vi "Data Logger Main.vi"(0 "WebDAV Push":bool, 1 "In Spec":bool[](array[boolean])=[FALSE, FALSE, FALSE, FALSE, FALSE, FALSE], 2 "Current Step":i32=2, 3 "Step Time Left":dbl=0.21101045608520508, 4 "Pump Data":T2={"Voltages"=[0.015201568603515625, 0.00335693359375, 0.003021240234375, 0.12260055541992188, 0.06085968017578125, 0.052234649658203125], "PumpCurrent"=[0.015201568603515625, 0.00335693359375, 0.003021240234375, 0.12260055541992188, 0.06085968017578125, 0.052234649658203125], "Speed"=[0.0, 0.0, 0.0, 0.0, 0.0, 0.0], "ControllerCurrent"=[0.015201568603515625, 0.00335693359375, 0.003021240234375, 0.12260055541992188, 0.06085968017578125, 0.052234649658203125], "Pressure"=[0.015201568603515625, 0.00335693359375, 0.003021240234375, 0.12260055541992188, 0.06085968017578125, 0.052234649658203125], "Flow"=[0.0, 0.0, 0.0, 0.125, 0.0625, 0.0625], "Elapsed Time (Display)"=[7.1, 7.1, 7.1, 458133.45, 458138.85000000003, 458126.75], "Avg Pressure"=0.0, "Avg Speed"=0.0, "Elapsed Time"=[4074.9003000000002, 4074.9003000000002, 4074.9003000000002, 4074.9003000000002, 4074.9003000000002, 4074.9003000000002]} {"Elapsed Time" format="%<%H:%M:%S>t"; "Elapsed Time (Display)" format="%<%H:%M:%S>t"; "Speed" format="%#_4f"; "ControllerCurrent" format="%#.1g"; "Pressure" format="%#.0f"; "Flow" format="%#.0f"; "PumpCurrent" format="%#.1g"; "Voltages" format="%#.0f"}, 5 "Tank Data":T1 {"PS Actual (V):" format="%.2f"; "Temp1" format="%#_2g"; "Temp2" format="%#_2g"}, 6 "Concat Data":bool, 7 "Record Time (sec)":dbl, 8 "Data Logger Mode":T8=enum."Main", 9 "Data Log Start":T3={"App Config"={"Location"="", "Profiles Path"=path "", "Current Profile"="", "CA Number"="", "Cycles Completed"=0, "Controller Type:"=enum."Kuhnke", "Stagger Time (ms)"=0, "Tank 1 Fuel"="", "Tank 2 Fuel"="", "Serial Numbers"={"Position 1 SN"="", "Position 2 SN"="", "Poaition 3 SN"="", "Position 4 SN"="", "Position 5 SN"="", "Position 6 SN"=""}, "Pumps Present"={"Pump 1"=FALSE, "Pump 2"=FALSE, "Pump 3"=FALSE, "Pump 4"=FALSE, "Pump 5"=FALSE, "Pump 6"=FALSE}, "VoltCtrlRef"="", "VoltageSelect"=FALSE, "Watlow Present"=FALSE, "Temp 1"=0.0, "Temp 2"=0.0, "V_Run PI?"=FALSE, "Voltage Limits"={"V_Step"=1e-05, "V_CmdMax"=0.0, "V_CmdMin"=0.0}, "Voltage Far PI"={"V_FarSlew"=10.0, "V_FarKp"=0.0, "V_FarKi"=0.0}, "Voltage Mid PI"={"V_MidSlew"=10.0, "V_MidKp"=0.0, "V_MidKi"=0.0}, "Voltage Close PI"={"V_CloseSlew"=10.0, "V_CloseKp"=0.0, "V_CloseKi"=0.0}, "Voltage Scale"={"V_FFm"=0.0, "V_FFb"=0.0}, "Voltage Cutoffs"={"V_MidCutoff"=0.0, "V_CloseCutoff"=0.0}, "Pressure Scale"={"Pres_FFm"=1e-05, "Pres_FFb"=0.0}, "Temp Format"=0, "Temp Tolerance"=0.0, "Target Voltage"=0.0, "Target Pressure"=0.0, "Data Log Init"={"Data Path"=path "", "Data Log Rate (S/s)"=0, "AKLH Rate (Hours/S)"=0.0, "Sync Time Offset (min)"=0, "IP Last 3"=0, "WebDAV IP"=""}, "Email Handler IP"="", "ADC Check"=FALSE, "3 Pump Tank"=FALSE, "Cycle Threshold:"=3.0, "Cycle Pts to Avg:"=3, "Anomaly Threshold:"=3.0, "Normal Steps:"=3, "Step Threshold:"=3.0, "Network Drive IP"="", "Network Drive Password"="", "Bank 1 Offset"=0.0, "Bank 2 Offset"=0.0}, "Profile"=[], "Controller Type"="", "Tank CMDs"={"PS CMD"=0.0, "Press CMD"=0.0, "Temp 1 CMD"=0.0, "Temp 2 CMD"=0.0}} {"App Config"."Bank 2 Offset" min=0.0 max=999999.0 step=1.0; "App Config"."Bank 1 Offset" min=0.0 max=999999.0 step=1.0; "App Config"."Step Threshold:" min=0.0 max=999999.0 step=1.0; "App Config"."Normal Steps:" max=999999 step=1; "App Config"."Anomaly Threshold:" min=0.0 max=999999.0 step=1.0; "App Config"."Cycle Pts to Avg:" max=999999 step=1; "App Config"."Cycle Threshold:" min=0.0 max=999999.0 step=1.0}, 11 "Data Log Init":T6) -> ()   [LabVIEW 2013]
uses:
  Data Logger Mode.ctl
  Data Log Init.ctl
  Data Log Start.ctl
  Type Defs/App Config.ctl
  Type Defs/Controller Names.ctl
  Controls/Tank CMDs.ctl
  Controls/Pump Data.ctl
  Controls/Tank Data.ctl
  <userlib>/_OpenG.lib/array/array.llb/Remove Duplicates from 1D Array (String)__ogtk.vi
  <userlib>/_OpenG.lib/array/array.llb/Filter 1D Array (String)__ogtk.vi
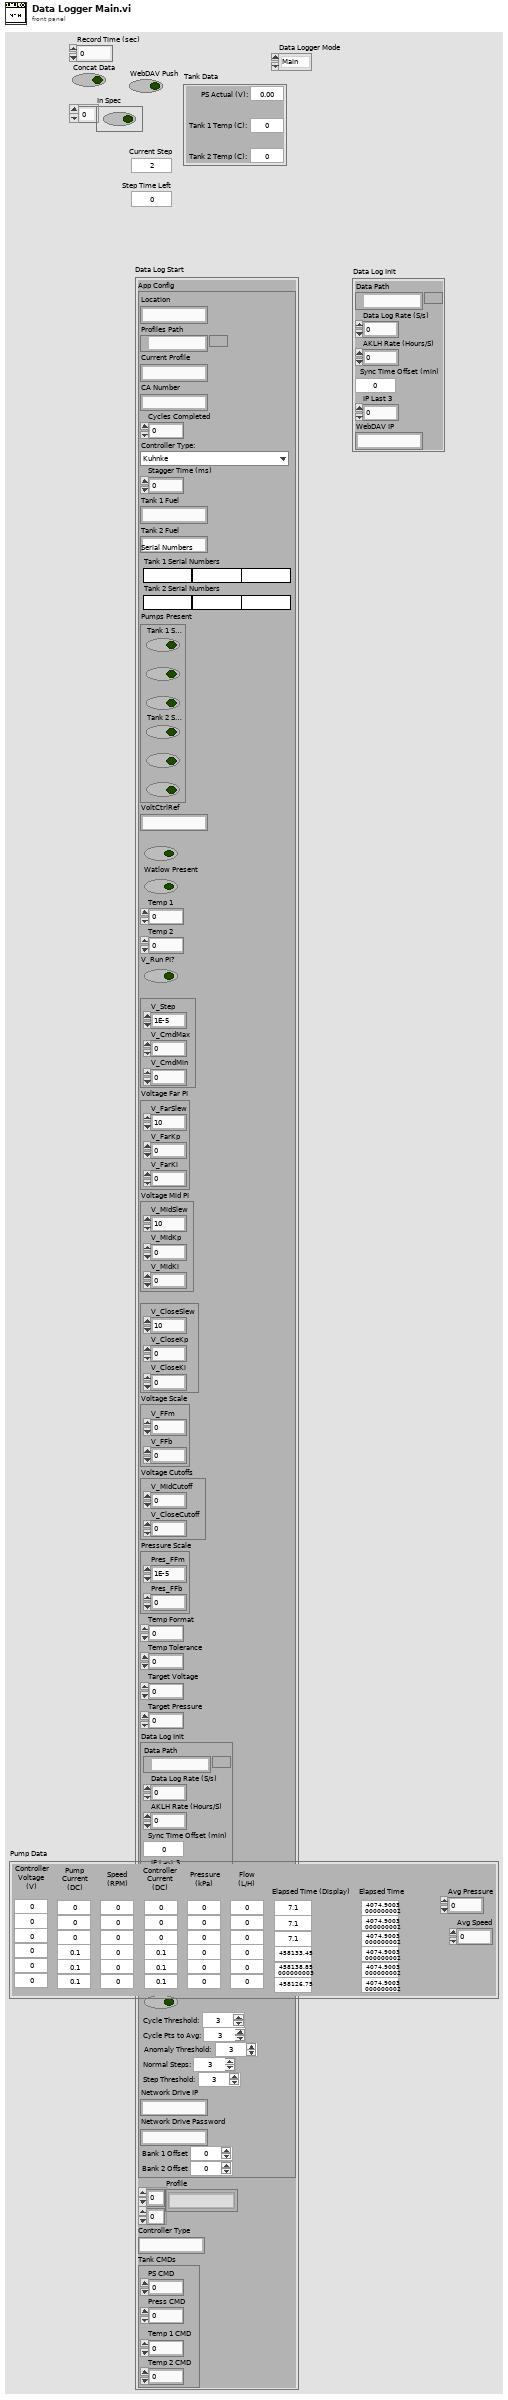
[diagram p1: front panel]
types:
  T1 = typedef "Tank Data.ctl" = cluster{"PS Actual (V):":dbl, "Temp1":dbl, "Temp2":dbl}
  T2 = typedef "Pump Data.ctl" = cluster{"Voltages":dbl[], "PumpCurrent":dbl[], "Speed":dbl[], "ControllerCurrent":dbl[], "Pressure":dbl[], "Flow":dbl[], "Elapsed Time (Display)":dbl[], "Avg Pressure":dbl, "Avg Speed":dbl, "Elapsed Time":dbl[]}
  T3 = typedef "Data Log Start.ctl" = cluster{"App Config":T4, "Profile":string[][], "Controller Type":string, "Tank CMDs":T7}
  T4 = typedef "App Config.ctl" = cluster{"Location":string, "Profiles Path":path, "Current Profile":string, "CA Number":string, "Cycles Completed":u32, "Controller Type:":T5, "Stagger Time (ms)":i32, "Tank 1 Fuel":string, "Tank 2 Fuel":string, "Serial Numbers":cluster{"Position 1 SN":string, "Position 2 SN":string, "Poaition 3 SN":string, "Position 4 SN":string, "Position 5 SN":string, "Position 6 SN":string}, "Pumps Present":cluster{"Pump 1":bool, "Pump 2":bool, "Pump 3":bool, "Pump 4":bool, "Pump 5":bool, "Pump 6":bool}, "VoltCtrlRef":string, "VoltageSelect":bool, "Watlow Present":bool, "Temp 1":dbl, "Temp 2":dbl, "V_Run PI?":bool, "Voltage Limits":cluster{"V_Step":dbl, "V_CmdMax":dbl, "V_CmdMin":dbl}, "Voltage Far PI":cluster{"V_FarSlew":dbl, "V_FarKp":dbl, "V_FarKi":dbl}, "Voltage Mid PI":cluster{"V_MidSlew":dbl, "V_MidKp":dbl, "V_MidKi":dbl}, "Voltage Close PI":cluster{"V_CloseSlew":dbl, "V_CloseKp":dbl, "V_CloseKi":dbl}, "Voltage Scale":cluster{"V_FFm":dbl, "V_FFb":dbl}, "Voltage Cutoffs":cluster{"V_MidCutoff":dbl, "V_CloseCutoff":dbl}, "Pressure Scale":cluster{"Pres_FFm":dbl, "Pres_FFb":dbl}, "Temp Format":i32, "Temp Tolerance":dbl, "Target Voltage":dbl, "Target Pressure":dbl, "Data Log Init":T6, "Email Handler IP":string, "ADC Check":bool, "3 Pump Tank":bool, "Cycle Threshold:":dbl, "Cycle Pts to Avg:":i32, "Anomaly Threshold:":dbl, "Normal Steps:":u32, "Step Threshold:":dbl, "Network Drive IP":string, "Network Drive Password":string, "Bank 1 Offset":dbl, "Bank 2 Offset":dbl}
  T5 = typedef "Controller Names.ctl" = enum16{"Kuhnke", "Helbako BLDC", "Conti", "Hella BLDC OL PWM", "Hella BLDC Turbine OL PWM", "Hella BLDC Pressure", "Helbako (old)", "TI PWM", "PSA", "Hella Gas", "Hella Diesel", "8 Comm", "10 Comm", "8 Comm Hella", "10 Comm Hella", "8 Comm Omron", "10 Comm Omron", "8 Comm Nissan", "10 Comm Nissan"}
  T6 = typedef "Data Log Init.ctl" = cluster{"Data Path":path, "Data Log Rate (S/s)":u32, "AKLH Rate (Hours/S)":dbl, "Sync Time Offset (min)":i32, "IP Last 3":i32, "WebDAV IP":string}
  T7 = typedef "Tank CMDs.ctl" = cluster{"PS CMD":dbl, "Press CMD":dbl, "Temp 1 CMD":dbl, "Temp 2 CMD":dbl}
  T8 = typedef "Data Logger Mode.ctl" = enum16{"Init", "Main", "Start", "Stop"}
  T9 = cluster{"Pump 1":bool, "Pump 2":bool, "Pump 3":bool, "Pump 4":bool, "Pump 5":bool, "Pump 6":bool}
  T10 = cluster{"Data Log Base":path, "AKLH Base":path, "AKLH Today Base":path, "AKLH Sync Base":path, "Data Log Rate (ms)":u32, "AKLH Rate (ms)":u32, "Sync Time (min)":i32, "Profile":string[][], "Target Speeds":string[], "App Config":T4, "AKLH Filenames":string[], "Data Log Dirs":path[], "AKLH Dirs":path[], "AKLH Today Dirs":path[], "AKLH Sync Dirs":path[], "Data Log Hdr Paths":path[], "AKLH Today Hdr Paths":path[], "Log Data":bool, "Data Log Times":u32[], "AKLH Log Times":u32[][], "WebDAV IP":string, "Tank CMDs":T7}
  T11 = cluster{"Position 1 SN":string, "Position 2 SN":string, "Poaition 3 SN":string, "Position 4 SN":string, "Position 5 SN":string, "Position 6 SN":string}
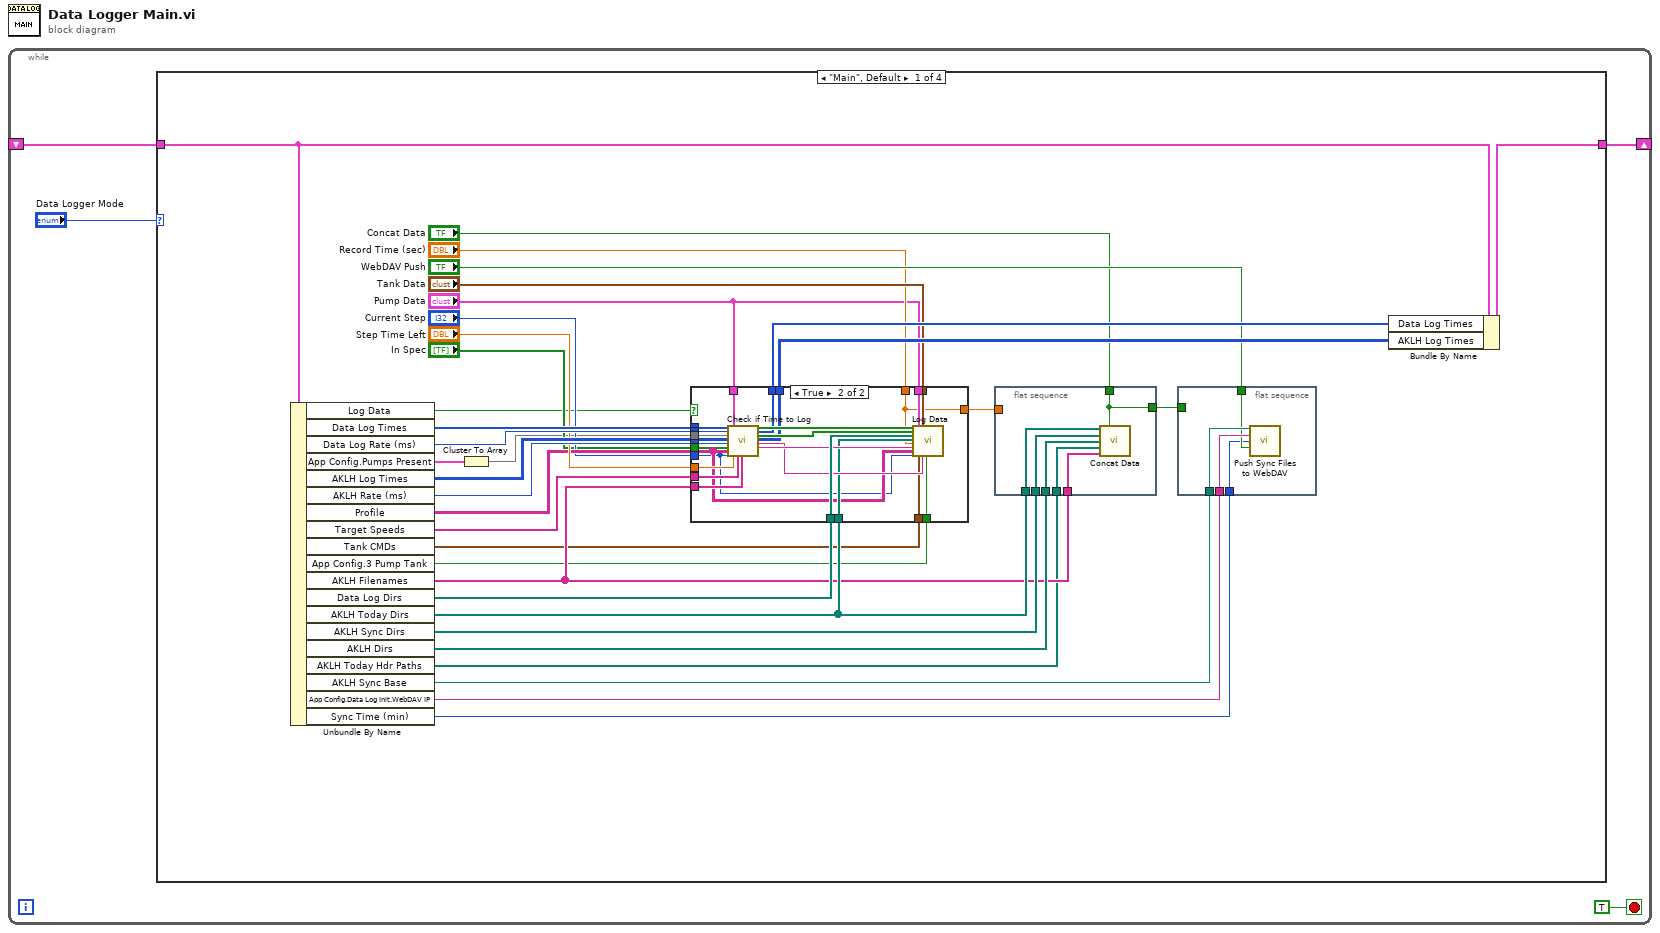
[diagram p0: block diagram]
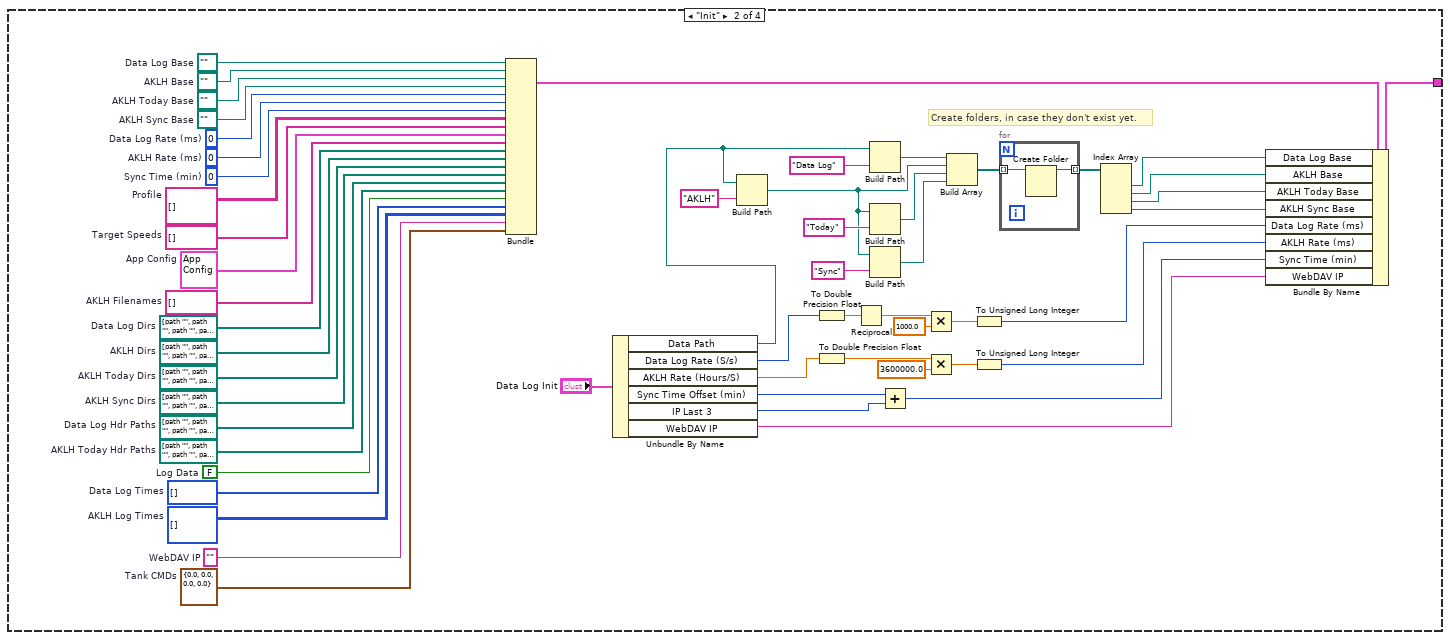
[diagram p3: hidden frame]
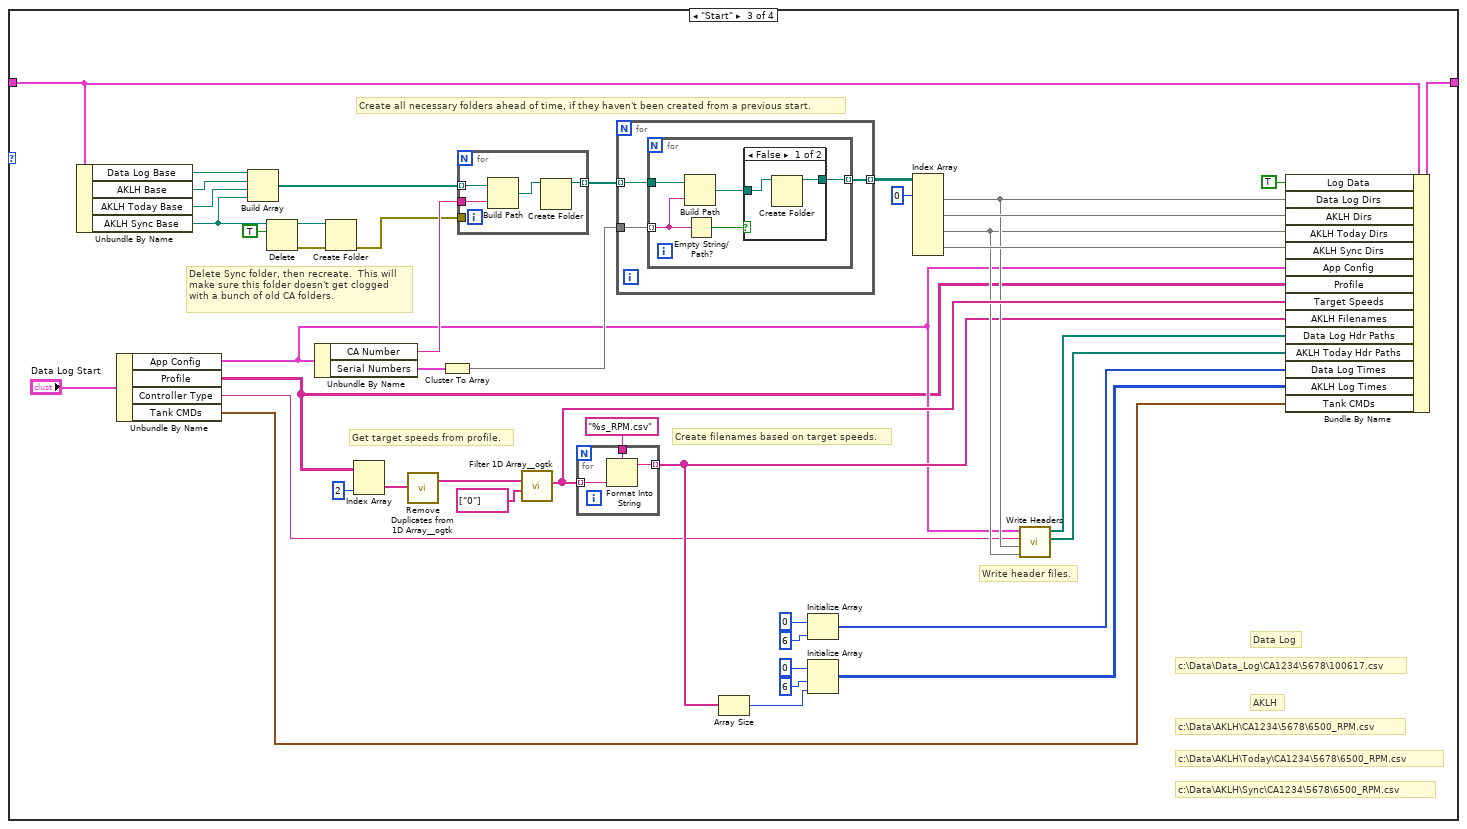
[diagram p4: hidden frame]
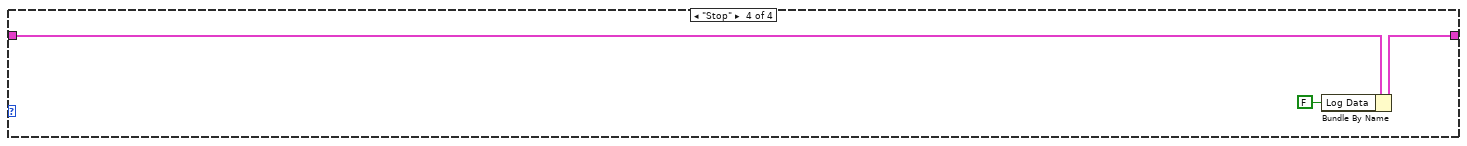
[diagram p6: hidden frame]
diagram:
  n1 = while {
    shift-right: [w2] -> _
    shift-left: _ -> [w1]
    stop <- TRUE stop-if-true
    n2 = case shown="\"Main\", Default" "Data Logger Mode" {
      tunnel: [w37 w124 w161 w196] -> w2
      tunnel: w1 -> [w38 _ w162 w197]
      frame "Main", Default {
        n3 = Unbundle By Name(w38) -> ("Log Data"=w9:bool, "Data Log Times"=w36:u32[], "Data Log Rate (ms)"=w35:u32, "App Config.Pumps Present"=w13:T9, "AKLH Log Times"=w34:u32[][], "AKLH Rate (ms)"=w33:u32, "Profile"=w18:string[][], "Target Speeds"=w31:string[], "Tank CMDs"=w16:T7, "App Config.3 Pump Tank"=w6:bool, "AKLH Filenames"=w24:string[], "Data Log Dirs"=w30:path[], "AKLH Today Dirs"=w27:path[], "AKLH Sync Dirs"=w26:path[], "AKLH Dirs"=w25:path[], "AKLH Today Hdr Paths"=w23:path[], "AKLH Sync Base"=w22:path, "App Config.Data Log Init.WebDAV IP"=w21:string, "Sync Time (min)"=w20:i32)
        n4 = Cluster To Array(cluster=w13) -> (array=w12:bool[])
        n5 = case shown="True" w9 {
          tunnel: w36 -> [w51 w76]
          tunnel: w35 -> [_ w75]
          tunnel: w34 -> [w50 w74]
          tunnel: w33 -> [_ w73]
          tunnel: "Step Time Left" -> [_ w72]
          tunnel: w31 -> [_ w71]
          tunnel: w30 -> [_ w68]
          tunnel: [w51 w65] -> w29
          tunnel: [w50 w64] -> w28
          tunnel: w27 -> [_ w63]
          tunnel: w24 -> [_ w62]
          tunnel: w18 -> [_ w56]
          tunnel: "Current Step" -> [_ w55]
          tunnel: w16 -> [_ w61]
          tunnel: "Tank Data" -> [_ w60]
          tunnel: "Pump Data" -> [_ w59]
          tunnel: "In Spec" -> [_ w58]
          tunnel: w12 -> [_ w57]
          tunnel: "Record Time (sec)" -> [w49 w54]
          tunnel: [w49 w54] -> w7
          tunnel: w6 -> [_ w53]
          tunnel: "Pump Data" -> [_ w52]
          frame False {
          }
          frame True {
            n6 = call "Check if Time to Log.vi"("Data Log Times IN"=w76, "Data Log Rate (ms)"=w75, "Pumps Present"=w57, "AKLH Log Times IN"=w74, "AKLH Rate (ms)"=w73, "In Spec"=w58, "Profile"=w56, "Current Step"=w55, "Pump Data"=w52, "Step Time Left"=w72, "Target Speeds"=w71, "AKLH Filenames"=w62) -> ("Log Data"=w70:bool[], "Data Log Times OUT"=w65:u32[], "Log AKLH"=w69:bool[], "AKLH Log Times OUT"=w64:u32[][], "AKLH Filename"=w66:string, "Target Speed"=w67:string)  [unwired: 10 in]
            n7 = call "Log Data.vi"("Log Data"=w70, "Log AKLH"=w69, "Data Log Dirs"=w68, "AKLH Today Dirs"=w63, "Record Time (sec)"=w54, "Target Speed"=w67, "Profile"=w56, "Current Step"=w55, "Pump Data"=w59, "Tank CMDs"=w61, "Tank Data"=w60, "AKLH Filename"=w66, "3 Pump Tank"=w53) -> ()  [unwired: 15 in]
          }
        }
        n8 = flat-sequence {
          tunnel: w27 -> [w48]
          tunnel: w26 -> [w47]
          tunnel: w25 -> [w46]
          tunnel: w24 -> [w45]
          tunnel: w23 -> [w44]
          tunnel: "Concat Data" -> [w43]
          tunnel: [w43] -> w8
          tunnel: w7 -> [_]
          frame #0 {
            n9 = call "Concat Data.vi"("AKLH Today Dirs"=w48, "Concat Data"=w43, "AKLH Sync Dirs"=w47, "AKLH Dirs"=w46, "AKLH Today Hdr Paths"=w44, "AKLH Filenames"=w45) -> ()  [unwired: 10 in]
          }
        }
        n10 = flat-sequence {
          tunnel: w22 -> [w42]
          tunnel: w21 -> [w41]
          tunnel: w20 -> [w39]
          tunnel: "WebDAV Push" -> [w40]
          tunnel: w8 -> [_]
          frame #0 {
            n11 = call "Push Sync Files to WebDAV.vi"("AKLH Sync Base"=w42, "WebDAV IP"=w41, "Sync Time (min)"=w39, "WebDAV Push"=w40) -> ()  [unwired: 12 in]
          }
        }
        n12 = Bundle By Name(cluster=w38, "Data Log Times"=w29, "AKLH Log Times"=w28) -> (w37:T10)
      }
      frame "Init" {
        w88 = T7 {"PS CMD"=0.0, "Press CMD"=0.0, "Temp 1 CMD"=0.0, "Temp 2 CMD"=0.0}  # Tank CMDs
        w94 = ""  # WebDAV IP
        w95 = u32[][] []  # AKLH Log Times
        w96 = u32[] []  # Data Log Times
        w97 = FALSE  # Log Data
        w98 = path[] [path "", path "", path "", path "", path "", path ""]  # AKLH Today Hdr Paths
        w99 = path[] [path "", path "", path "", path "", path "", path ""]  # Data Log Hdr Paths
        w100 = path[] [path "", path "", path "", path "", path "", path ""]  # AKLH Sync Dirs
        w101 = path[] [path "", path "", path "", path "", path "", path ""]  # AKLH Today Dirs
        w102 = path[] [path "", path "", path "", path "", path "", path ""]  # AKLH Dirs
        w103 = path[] [path "", path "", path "", path "", path "", path ""]  # Data Log Dirs
        w104 = string[] []  # AKLH Filenames
        w105 = T4 {"Location"="", "Profiles Path"=path "", "Current Profile"="", "CA Number"="", "Cycles Completed"=0, "Controller Type:"=enum."Kuhnke", "Stagger Time (ms)"=0, "Tank 1 Fuel"="", "Tank 2 Fuel"="", "Serial Numbers"={"Position 1 SN"="", "Position 2 SN"="", "Poaition 3 SN"="", "Position 4 SN"="", "Position 5 SN"="", "Position 6 SN"=""}, "Pumps Present"={"Pump 1"=FALSE, "Pump 2"=FALSE, "Pump 3"=FALSE, "Pump 4"=FALSE, "Pump 5"=FALSE, "Pump 6"=FALSE}, "VoltCtrlRef"="", "VoltageSelect"=FALSE, "Watlow Present"=FALSE, "Temp 1"=0.0, "Temp 2"=0.0, "V_Run PI?"=FALSE, "Voltage Limits"={"V_Step"=0.0, "V_CmdMax"=0.0, "V_CmdMin"=0.0}, "Voltage Far PI"={"V_FarSlew"=0.0, "V_FarKp"=0.0, "V_FarKi"=0.0}, "Voltage Mid PI"={"V_MidSlew"=0.0, "V_MidKp"=0.0, "V_MidKi"=0.0}, "Voltage Close PI"={"V_CloseSlew"=0.0, "V_CloseKp"=0.0, "V_CloseKi"=0.0}, "Voltage Scale"={"V_FFm"=0.0, "V_FFb"=0.0}, "Voltage Cutoffs"={"V_MidCutoff"=0.0, "V_CloseCutoff"=0.0}, "Pressure Scale"={"Pres_FFm"=0.0, "Pres_FFb"=0.0}, "Temp Format"=0, "Temp Tolerance"=0.0, "Target Voltage"=0.0, "Target Pressure"=0.0, "Data Log Init"={"Data Path"=path "", "Data Log Rate (S/s)"=0, "AKLH Rate (Hours/S)"=0.0, "Sync Time Offset (min)"=0, "IP Last 3"=0, "WebDAV IP"=""}, "Email Handler IP"="", "ADC Check"=FALSE, "3 Pump Tank"=FALSE, "Cycle Threshold:"=0.0, "Cycle Pts to Avg:"=0, "Anomaly Threshold:"=0.0, "Normal Steps:"=0, "Step Threshold:"=0.0, "Network Drive IP"="", "Network Drive Password"="", "Bank 1 Offset"=0.0, "Bank 2 Offset"=0.0}  # App Config
        w107 = string[][] []  # Profile
        w106 = string[] []  # Target Speeds
        w109 = 0  # Sync Time (min)
        w126 = u32 0  # AKLH Rate (ms)
        w127 = u32 0  # Data Log Rate (ms)
        w128 = path ""  # AKLH Sync Base
        w129 = path ""  # AKLH Today Base
        w130 = path ""  # AKLH Base
        w131 = path ""  # Data Log Base
        # "Create folders, in case they don't exist yet."
        n13 = Bundle("Data Log Base"=w131, "AKLH Base"=w130, "AKLH Today Base"=w129, "AKLH Sync Base"=w128, "Data Log Rate (ms)"=w127, "AKLH Rate (ms)"=w126, "Sync Time (min)"=w109, "Profile"=w107, "Target Speeds"=w106, "App Config"=w105, "AKLH Filenames"=w104, "Data Log Dirs"=w103, "AKLH Dirs"=w102, "AKLH Today Dirs"=w101, "AKLH Sync Dirs"=w100, "Data Log Hdr Paths"=w99, "AKLH Today Hdr Paths"=w98, "Log Data"=w97, "Data Log Times"=w96, "AKLH Log Times"=w95, "WebDAV IP"=w94, "Tank CMDs"=w88) -> (w125:T10)  [unwired: 1 in]
        n14 = Unbundle By Name("Data Log Init") -> ("Data Path"=w89:path, "Data Log Rate (S/s)"=w84:u32, "AKLH Rate (Hours/S)"=w79:dbl, "Sync Time Offset (min)"=w90:i32, "IP Last 3"=w91:i32, "WebDAV IP"=w92:string)
        n15 = Build Path(base path=w89, name or relative path="AKLH") -> (appended path=w118:path)
        n16 = To Double Precision Float(number=w84) -> (double precision float=w87:dbl)
        n17 = To Double Precision Float(number=w79) -> (double precision float=w78:dbl)
        n18 = Reciprocal(x=w87) -> (1/x=w86:dbl)
        n19 = Build Path(base path=w89, name or relative path="Data Log") -> (appended path=w119:path)
        n20 = Build Path(base path=w118, name or relative path="Today") -> (appended path=w117:path)
        n21 = Build Path(base path=w118, name or relative path="Sync") -> (appended path=w116:path)
        n22 = Add(x=w90, y=w91) -> (x+y=w108:i32)
        n23 = Multiply(x=w86, y=1000.0) -> (x*y=w83:dbl)
        n24 = Multiply(x=w78, y=3600000.0) -> (x*y=w81:dbl)
        n25 = Build Array(w119, w118, w117, w116) -> (w115:path[])
        n26 = To Unsigned Long Integer(number=w83) -> (unsigned 32bit integer=w82:u32)
        n27 = To Unsigned Long Integer(number=w81) -> (unsigned 32bit integer=w77:u32)
        n28 = for {
          tunnel: w115 -> [w133] mode=indexing
          tunnel: [w132] -> w114 mode=indexing
          n29 = Create Folder(path (use dialog)=w133) -> (created path=w132:path)  [unwired: 2 in, 2 out]
        }
        n30 = Index Array(array=w114) -> (element #1=w113:path, element #2=w112:path, element #3=w111:path, element #4=w110:path)  [unwired: 4 in]
        n31 = Bundle By Name(cluster=w125, "Data Log Base"=w113, "AKLH Base"=w112, "AKLH Today Base"=w111, "AKLH Sync Base"=w110, "Data Log Rate (ms)"=w82, "AKLH Rate (ms)"=w77, "Sync Time (min)"=w108, "WebDAV IP"=w92) -> (w124:T10)
      }
      frame "Start" {
        # "Delete Sync folder, then recreate.  This will\nmake sure this folder doesn't get clogged \nwith a bunch of old CA folders."
        # "Write header files."
        # "Create filenames based on target speeds."
        # "Get target speeds from profile."
        # "Create all necessary folders ahead of time, if they haven't been created from a previous start."
        # "c:\\Data\\AKLH\\Sync\\CA1234\\5678\\6500_RPM.csv"
        # "c:\\Data\\AKLH\\Today\\CA1234\\5678\\6500_RPM.csv"
        # "c:\\Data\\AKLH\\CA1234\\5678\\6500_RPM.csv"
        # "AKLH"
        # "Data Log"
        # "c:\\Data\\Data_Log\\CA1234\\5678\\100617.csv"
        n32 = Unbundle By Name(w162) -> ("Data Log Base"=w170:path, "AKLH Base"=w169:path, "AKLH Today Base"=w168:path, "AKLH Sync Base"=w138:path)
        n33 = Unbundle By Name("Data Log Start") -> ("App Config"=w143:T4, "Profile"=w142:string[][], "Controller Type"=w141:string, "Tank CMDs"=w140:T7)
        n34 = Build Array(w170, w169, w168, w138) -> (w167:path[])
        n35 = Delete(path (use dialog)=w138, entire hierarchy (F)=TRUE) -> (deleted path=w136:path, error out=w135:errorcluster)  [unwired: 3 in, 1 out]
        n36 = Unbundle By Name(w143) -> ("CA Number"=w166:string, "Serial Numbers"=w174:T11)
        n37 = Create Folder(path (use dialog)=w136, error in=w135) -> (error out=w134:errorcluster)  [unwired: 1 in, 2 out]
        n38 = Index Array(array=w142, index (col)=2 ("disabled index (col)")) -> (element=w175:string[])  [unwired: 1 in]
        n39 = call-poly <userlib>:"Remove Duplicates from 1D Array__ogtk.vi"("Input Array"=w175) -> ("Output Array"=w171:string[])  [unwired: 1 out]
        n40 = Cluster To Array(cluster=w174) -> (array=w173:string[])
        n41 = for {
          tunnel: w167 -> [w183] mode=indexing
          tunnel: [w181] -> w165 mode=indexing
          tunnel: w166 -> [w180]
          tunnel: w134 -> [_]
          n42 = Build Path(base path=w183, name or relative path=w180) -> (appended path=w182:path)
          n43 = Create Folder(path (use dialog)=w182) -> (created path=w181:path)  [unwired: 2 in, 2 out]
        }
        n44 = call-poly <userlib>:"Filter 1D Array__ogtk.vi"("items to filter"=string[] ["0"], "array"=w171) -> ("filtered array"=w158:string[])  [unwired: 4 in, 1 out]
        n45 = for {
          tunnel: w158 -> [w179] mode=indexing
          tunnel: "%s_RPM.csv" ("format string") -> [w178]
          tunnel: [w177] -> w147 mode=indexing
          n46 = Format Into String(format string=w178, w179) -> (resulting string=w177:string)  [unwired: 2 in, 1 out]
        }
        n47 = for {
          tunnel: w165 -> [w185] mode=indexing
          tunnel: w173 -> [w186]
          tunnel: [w184] -> w164 mode=indexing
          n48 = for {
            tunnel: w186 -> [w190] mode=indexing
            tunnel: w185 -> [w191]
            tunnel: [w187] -> w184 mode=indexing
            n49 = Build Path(base path=w191, name or relative path=w190) -> (appended path=w188:path)
            n50 = Empty String/Path?(string/path=w190) -> (empty?=w189:bool)
            n51 = case shown="False" w189 {
              tunnel: w188 -> [w193 w194]
              tunnel: [w192 w194] -> w187
              frame False {
                n52 = Create Folder(path (use dialog)=w193) -> (created path=w192:path)  [unwired: 2 in, 2 out]
              }
              frame True {
              }
            }
          }
        }
        n53 = Array Size(array=w147) -> (size(s)=w146:i32)
        n54 = Initialize Array(u32 0, 6 ("dimension size")) -> (w150:u32[])
        n55 = Initialize Array(u32 0, 6 ("dimension size"), w146) -> (w145:u32[][])
        n56 = Index Array(array=w164, index (row) #1=0 ("disabled index (col)")) -> (element #1=w157:path[], element #2=w160:path[], element #3=w156:path[], element #4=w159:path[])  [unwired: 7 in]
        n57 = call "Write Headers.vi"("AKLH Today Dirs"=w156, "Data Log Dirs"=w157, "Controller Type"=w141, "App Config"=w143) -> ("AKLH Today Header Paths"=w154:path[], "Data Log Header Paths"=w155:path[])  [unwired: 6 in]
        n58 = Bundle By Name(cluster=w162, "Log Data"=TRUE, "Data Log Dirs"=w157, "AKLH Dirs"=w160, "AKLH Today Dirs"=w156, "AKLH Sync Dirs"=w159, "App Config"=w143, "Profile"=w142, "Target Speeds"=w158, "AKLH Filenames"=w147, "Data Log Hdr Paths"=w155, "AKLH Today Hdr Paths"=w154, "Data Log Times"=w150, "AKLH Log Times"=w145, "Tank CMDs"=w140) -> (w161:T10)
      }
      frame "Stop" {
        n59 = Bundle By Name(cluster=w197, "Log Data"=FALSE) -> (w196:T10)
      }
    }
  }
